vi "Read Motion Profile Array.vi"(8 "error in (no error)":errorcluster, 11 "Motion Profile Generator in":refnum<class "Motion Profile Generator.lvclass">) -> (0 "error out":errorcluster, 2 "Motion Profile Array":T1[](array[typedef]), 3 "Motion Profile Generator out":refnum<class "Motion Profile Generator.lvclass">)   [LabVIEW 2019, in "Motion Profile Generator.lvclass"]
uses:
  Motion Profile Generator.lvclass
  Type Defs/Motion Profile Point.ctl
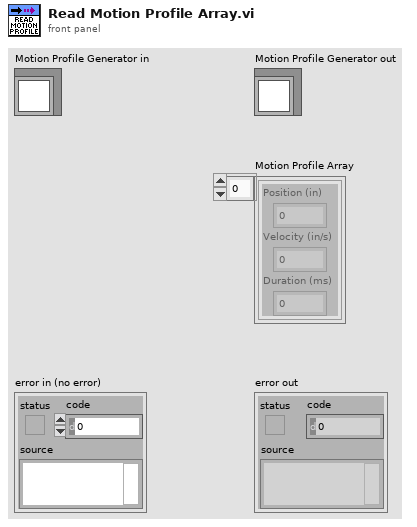
[diagram p1: front panel]
types:
  T1 = typedef "Motion Profile Generator.lvclass/Motion Profile Point.ctl" = cluster{"Position (in)":dbl, "Velocity (in/s)":dbl, "Duration (ms)":dbl}
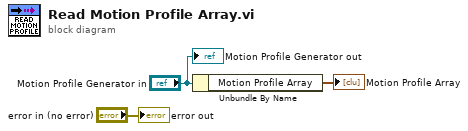
[diagram p0: block diagram]
diagram:
  n1 = Unbundle By Name("Motion Profile Generator in") -> ("Motion Profile Array"=→"Motion Profile Array":T1[])
  "error out" <- "error in (no error)"
  "Motion Profile Generator out" <- "Motion Profile Generator in"
